vi "Start Group.vi"(8 "Error In":errorcluster, 10 "Style Sheet":string, 11 "Front Panel Objects":refnum<vi>[](array[refnum])) -> (0 "Error Out":errorcluster)   [LabVIEW 2019, in "LSS.lvlib"]
doc: "Creates groupings of objects based on the Style Sheet input. All styles applied to the group itself will apply to all objects of the group.\nGroupings must be started before tags are marked into controls. Otherwise the groups will not be marked into the tag hierarchy properly.\nThere can be any number of groups, but each control can presently only belong to one group.\n\n<b>Inputs:</b>\n<b>Front Panel Objects</b> - Contains array of all objects on the front panel.\n<b>Style Sheet</b> - Style sheet determining how objects will be grouped. The format of the style sheet for grouping objects is as follows:\ngrouping{\n objectGroupName:frontPanelObjectName;\n objectGroupName2:frontPanelObjectName2;\n}\nWhere the specifier grouping must stay the same. objectGroupName is the name of the group, for example \"Group 1\". frontPanelObjectName is the name of the item on the front panel, for example \"Stop Button\". To add two buttons to group alpha would look as follows:\ngrouping{\n group alpha:Start Button;\n group alpha:Stop Button;\n}\n<b>Error In</b> - Standard Error In terminal\n\n<b>Outputs:</b>\n<b>Error Out</b> - Standard Error out terminal"
uses:
  LSS.lvlib
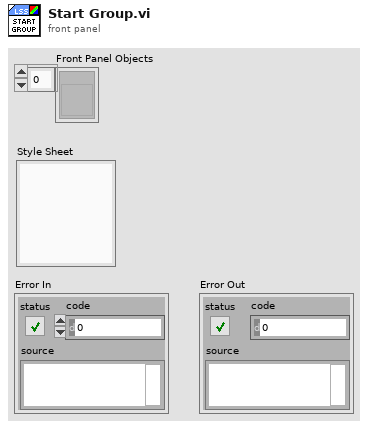
[diagram p1: front panel]
types:
  T1 = typedef "LSS.lvlib/Style.ctl" = cluster{"Specifier":string, "Properties":cluster{"Property":string, "Value":string}[]}
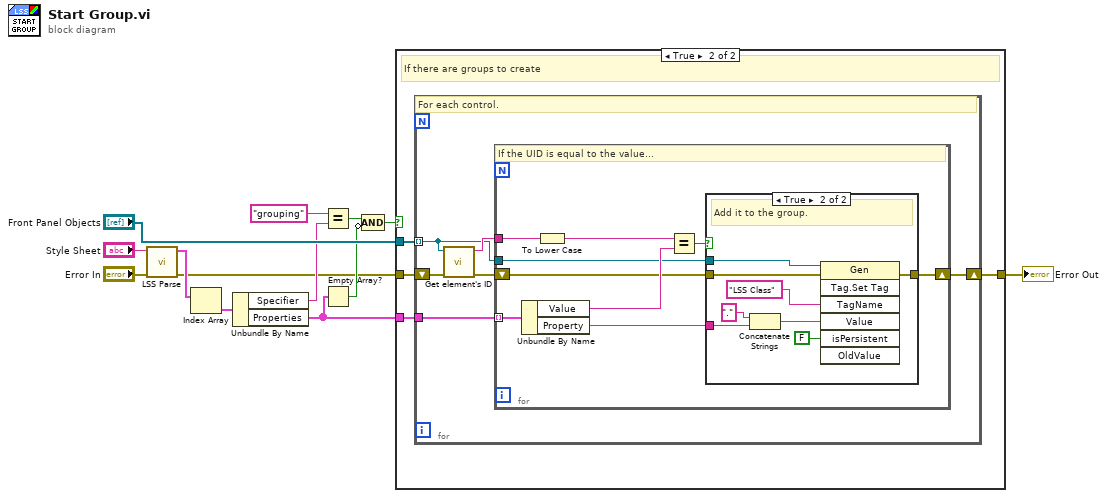
[diagram p0: block diagram]
diagram:
  n1 = call "LSS Parse.vi"("Error in"="Error In", "Style Sheet"="Style Sheet") -> ("Error out"=w2:errorcluster, "LSS Styles"=w12:T1[])  [unwired: 8 in]
  n2 = Index Array(array=w12) -> (element=w10:T1)  [unwired: 1 in]
  n3 = Unbundle By Name(w10) -> ("Specifier"=w7:string, "Properties"=w9:cluster{"Property":string, "Value":string}[])
  n4 = Equal?(x="grouping", y=w7) -> (x = y?=w5:bool)
  n5 = Empty Array?(array=w9) -> (empty?=w8:bool)
  n6 = Compound Arithmetic op=AND(w5, invert w8) -> (w4:bool)
  n7 = case shown="True" w4 {
    tunnel: w9 -> [_ w17]
    tunnel: "Front Panel Objects" -> [_ w18]
    tunnel: w2 -> [w14 w16]
    tunnel: [w14 w15] -> w1
    frame False {
      # "There are no groups to create, do nothing."
    }
    frame True {
      # "If there are groups to create"
      n8 = for {
        tunnel: w18 -> [w22] mode=indexing
        tunnel: w17 -> [w24]
        shift-right: [w19] -> w15
        shift-left: w16 -> [w21]
        # "For each control."
        n9 = call "Get element's ID.vi"("Error in"=w21, "GObject in"=w22) -> ("Error out"=w20:errorcluster, "ID"=w23:string)  [unwired: 8 in]
        n10 = for {
          tunnel: w24 -> [w33] mode=indexing
          tunnel: w23 -> [w32]
          tunnel: w22 -> [w29]
          shift-right: [w26] -> w19
          shift-left: w20 -> [w27]
          # "If the UID is equal to the value..."
          n11 = Unbundle By Name(w33) -> ("Value"=w31:string, "Property"=w28:string)
          n12 = To Lower Case(string=w32) -> (all lower case string=w25:string)
          n13 = Equal?(x=w25, y=w31) -> (x = y?=w30:bool)
          n14 = case shown="True" w30 {
            tunnel: w29 -> [_ w42]
            tunnel: w28 -> [_ w39]
            tunnel: w27 -> [w34 w36]
            tunnel: [w34 w35] -> w26
            frame False {
              # "do nothing if not part of group."
            }
            frame True {
              # "Add it to the group."
              n15 = Concatenate Strings("." ("string"), w39) -> (w38:string)
              n16 = invoke class="Gen" method="Tag.Set Tag"(reference=w42, error in=w36, "TagName"="LSS Class" ("Tag Name"), "Value"=w38, "isPersistent"=FALSE ("Is Persistent?")) -> (error out=w35:errorcluster)  [unwired: 2 in, 6 out]
            }
          }
        }
      }
    }
  }
  "Error Out" <- w1
